vi "LDA_meas_global_2.vi"() -> ()   [LabVIEW 2015]
uses:
  Controls/BSA_info_Cluster.ctl
panel:
  in  "Probe Type 2":string
  in  "Wavelength 2 (nm)":dbl=514.5 format="%.1f"
  in  "Beams Colour 2":string(combo)
  in  "Focal Length 2 (mm)":dbl
  in  "Beam Separation 2 (mm)":dbl
  in  "LDA 1st Group":dbl[][](array[numeric])
  in  "Vel LDA2 Non Coincident":dbl[](array[numeric]) format="%.2f"
  in  "Arrival times LDA2":dbl[](array[numeric]) format="%.2f"
  in  "Transit times LDA2":dbl[](array[numeric]) format="%.2f"
  in  "LDA 2nd Group":dbl[][](array[numeric])
  in  "Additional BSA2 Setup":string
  in  "Max Record length BSA2":dbl=2.0 format="%.2f"
  out "Max Vel BSA2":dbl=1.8339999999999999 format="%.2f"
  out "Min Vel BSA2":dbl=-1.8339999999999999 format="%.2f"
  out "High Volt BSA2":i16=1896 min=0 max=2040 step=8
  out "Signal gain BSA2":i16=32 min=0 max=57 step=1
  in  "Buffer mode":enum16{"One shot", "Ring", "FIFO"}(ring)
  out "Optic Calib factor BSA2":dbl=3.668 format="%.4e"
  in  "Multiply Velocity by -1":bool
  out "Vel Comp BSA2":string="W"
  in  "Slippage info":string
  out "BSA2 info":T1={"GPIB Address"="13", "No of Check Bytes"=4, "Extra Info"="57N11", "COLOUR"=52224, "Wavelength (nm)"=52224.0} {"Wavelength (nm)" format="%.1f"}
  in  "data type":T2(array[ring])=[enum."Velocity", enum."Arrival time"]
  in  "Number of measured quantities":i32=2
  in  "Bandwidth BSA2":dbl=3.668 format="%.2f"
  in  "Centre Freq BSA2":dbl format="%.2f"
  out "Anode current limit (mA)":T3(ring)=enum."0.1"
  in  "Record length BSA2":dbl=2.0 format="%.2f"
  out "Output":T4={"Output data format"=enum."Velocity, arrival time", "Non-validated signals"=enum."Accept"}
  out "Range":T5={"Centre frequency"=16, "Bandwidth"=10, "Units"=enum."m/s", "Frequency shift"=enum."Enabled"} {"Bandwidth" items=["3.877E-3", "7.754E-3", "15.508E-3", "31.016E-3", "62.031E-3", "124.063E-3", "248.125E-3", "496.250E-3", "992.500E-3", "1.985E+0", "3.970E+0", "7.940E+0", "15.880E+0", "31.760E+0"]; "Centre frequency" items=["-15.880E+0", "-14.888E+0", "-13.895E+0", "-12.902E+0", "-11.910E+0", "-10.918E+0", "-9.925E+0", "-8.933E+0", "-7.940E+0", "-6.947E+0", "-5.955E+0", "-4.963E+0", "-3.970E+0", "-2.978E+0", "-1.985E+0", "-992.500E-3", "0.000E+0", "992.500E-3", "1.985E+0", "2.978E+0", "3.970E+0", "4.963E+0", "5.955E+0", "6.947E+0", "7.940E+0", "8.933E+0", "9.925E+0", "10.918E+0", "11.910E+0", "12.902E+0", "13.895E+0", "14.888E+0", "15.880E+0"]}
  out "Analysis parameters":T6={"Burst criterion"=enum."Envelope", "Oversize reject level"=enum."1 (disabled)", "Pedestal attenuation"=enum."0", "Record length"=enum."32", "Quality factor"=0} {"Quality factor" min=0 max=80 step=10}
  out "Data collection mode":T7 {"Duty cycle (%)" format="%.2f"; "Dead time (s)" format="%.2f"}
  out "Clock parameters":T8={"Arrival time clock"=enum."Internal", "Clock source"=enum."Slave", "Coincidence"=enum."Slave"}
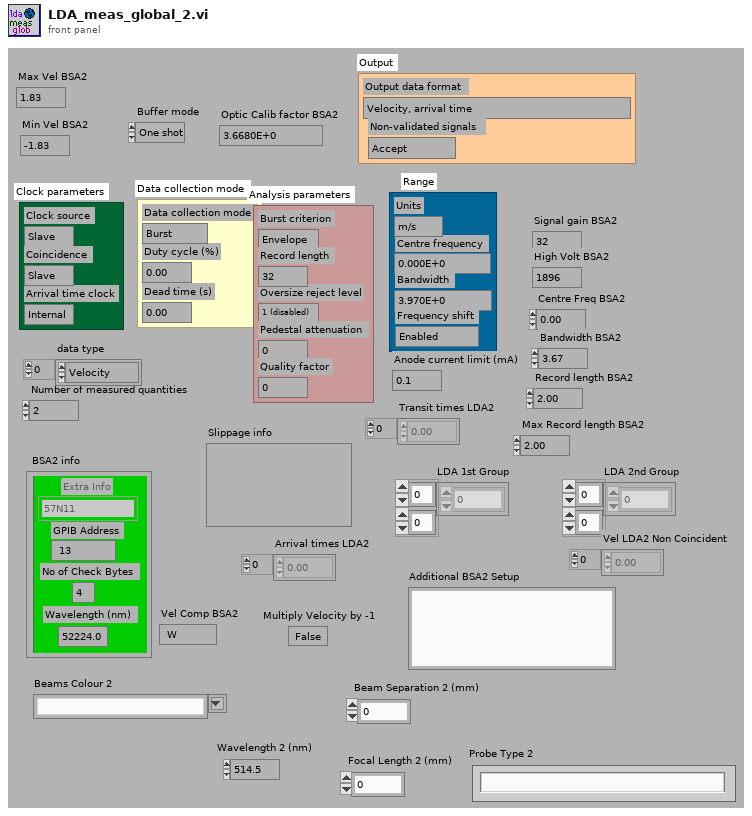
[diagram p1: front panel]
types:
  T1 = typedef "BSA_info_Cluster.ctl" = cluster{"GPIB Address":string, "No of Check Bytes":i32, "Extra Info":string, "COLOUR":u32, "Wavelength (nm)":dbl}
  T2 = enum16{"Velocity", "Transit time", "Arrival time"}[]
  T3 = enum16{"6.4", "3.2", "1.6", "0.8", "0.4", "0.2", "0.1", "0.05"}
  T4 = cluster{"Output data format":enum16{"Velocity, transit time, arrival time", "Velocity, arrival time", "Velocity, transit time", "Velocity"}, "Non-validated signals":enum16{"Accept", "Reject"}}
  T5 = cluster{"Centre frequency":u16, "Bandwidth":u16, "Units":enum16{"Hz", "m/s"}, "Frequency shift":enum16{"Disabled", "Enabled"}}
  T6 = cluster{"Burst criterion":enum16{"Envelope", "Pedestal", "Env and ped"}, "Oversize reject level":enum16{"1 (disabled)", "2", "3", "4", "5", "6", "7", "8", "9"}, "Pedestal attenuation":enum16{"0", "6", "12", "18"}, "Record length":enum16{"8", "16", "32", "64"}, "Quality factor":i16}
  T7 = cluster{"Dead time (s)":dbl, "Duty cycle (%)":dbl, "Data collection mode":enum16{"Burst", "Contiuous", "Dead time", "External"}}
  T8 = cluster{"Arrival time clock":enum16{"External", "Internal"}, "Clock source":enum16{"Slave", "Master", "Private"}, "Coincidence":enum16{"Slave", "Master", "Private"}}
diagram:
